vi "AddLogMsg.vi"(7 "LogLevel":T1=enum."None", 8 "error in (no error)":errorcluster, 10 "LogMsg":string) -> (0 "error out":errorcluster)   [LabVIEW 2018, in "Config_class.lvlib" / "Config.lvclass"]
uses:
  Config.lvclass
  Typedefs/eLogLvl.ctl
  Config.lvclass/Config.ctl
  Accessors/Read Logging.vi
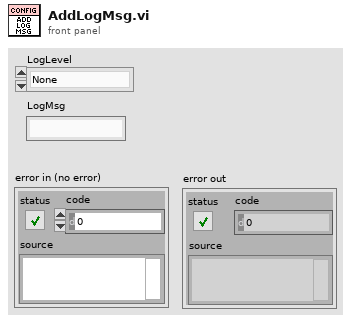
[diagram p1: front panel]
types:
  T1 = typedef "Config_class.lvlib/Config.lvclass/eLogLvl.ctl" = enum16{"Normal", "Verbose", "None"}
  T2 = typedef "Config_class.lvlib/Config.lvclass/Logging.ctl" = cluster{"eLogLvl":T1, "Log File Path":path, "btnLogFile":bool}
  T3 = enum16{"open", "replace", "create", "open or create", "replace or create", "replace or create with confirmation"}
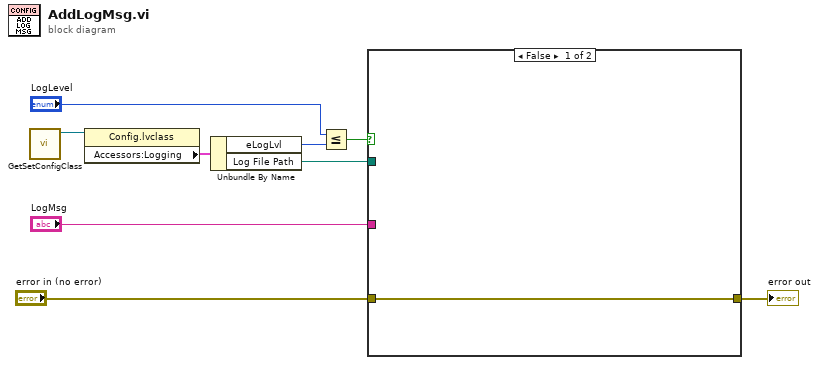
[diagram p0: block diagram]
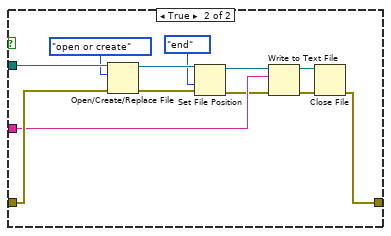
[diagram p2: hidden frame]
diagram:
  n1 = call "GetSetConfigClass.vi"() -> ("Ref out"=w9:refnum<class "Config.lvclass">)  [unwired: 11 in]
  n2 = property class="Config.lvclass"(reference=w9) -> ("Accessors:Logging"=w8:T2)  [unwired: 1 in, 2 out]
  n3 = Unbundle By Name(w8) -> ("eLogLvl"=w7:T1, "Log File Path"=w2:path)
  n4 = Less Or Equal?(x="LogLevel", y=w7) -> (x <= y?=w6:bool)
  n5 = case shown="False" w6 {
    tunnel: "error in (no error)" -> [w10 w18]
    tunnel: [w10 w11] -> w4
    tunnel: "LogMsg" -> [_ w16]
    tunnel: w2 -> [_ w22]
    frame False {
    }
    frame True {
      n6 = Open/Create/Replace File(file path (use dialog)=w22, error in=w18, operation (0:open)=T3."open or create") -> (refnum out=w20:refnum<file>, error out=w15:errorcluster)  [unwired: 3 in, 1 out]
      n7 = Set File Position(refnum=w20, from (0:start)=enum16{"start", "end", "current"}."end", error in=w15) -> (refnum out=w17:refnum<file>, error out=w14:errorcluster)  [unwired: 1 in]
      n8 = Write to Text File(file (use dialog)=w17, text=w16, error in=w14) -> (refnum out=w12:refnum<file>, error out=w13:errorcluster)  [unwired: 1 in, 1 out]
      n9 = Close File(refnum=w12, error in=w13) -> (error out=w11:errorcluster)  [unwired: 1 out]
    }
  }
  "error out" <- w4
